vi "CAN Single2Double.vi"(11 "Scale overall":sgl format="%.24g") -> (2 "Zahl":dbl format="%.20f", 3 "Numerisch":dbl format="%.24g")   [LabVIEW 2020, in "CAN Konfig.lvlib"]
uses:
  CAN Konfig.lvlib
panel:
  out "String in F-Format":string
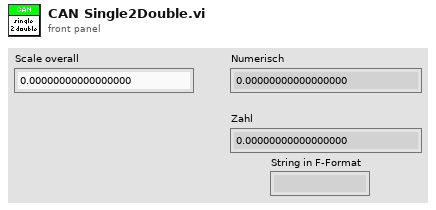
[diagram p1: front panel]
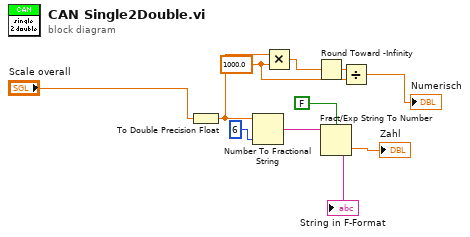
[diagram p0: block diagram]
diagram:
  w7 = 1000.0 ("y")
  n1 = To Double Precision Float(number="Scale overall") -> (double precision float=w6:dbl)
  n2 = Number To Fractional String(number=w6, precision (6)=i16 6 ("Genauigkeit (6)")) -> (F-format string=w9:string)  [unwired: 2 in]
  "String in F-Format" <- w9
  n3 = Multiply(x=w6, y=w7) -> (x*y=w2:dbl)
  n4 = Round Toward -Infinity(1:w2) -> (0:w3:dbl)
  n5 = Fract/Exp String To Number(use system decimal point (T)=FALSE ("Systemdezimalzeichen verwenden (T)"), string=w9) -> (number=→"Zahl":dbl)  [unwired: 2 in, 1 out]
  n6 = Divide(x=w3, y=w7) -> (x/y=→"Numerisch":dbl)
